vi "Best fit circle.vi"(0 "x array":dbl[](array[numeric]), 1 "y array":dbl[](array[numeric])) -> (2 "x centre":dbl, 3 "y centre":dbl, 4 "radius":dbl)   [LabVIEW 2014]
doc: "Finds the best fit circle using a least squares method. Input arrays (corresponding values of x and y) must have a minimum of 3 values each"
uses:
  <vilib>/Analysis/baseanly.llb/Real A x B.vi
  <vilib>/Analysis/baseanly.llb/A x Vector.vi
  <vilib>/Analysis/baseanly.llb/Real Inverse Matrix.vi
  <vilib>/Analysis/Matrix/Numeric/Conversions/Array To Matrix - RA2.vi
  <vilib>/Analysis/Matrix/NI_Matrix.lvlib
  <vilib>/Analysis/NI_AALBase.lvlib
panel:
  # "Paul Nathan 23/06/2015"
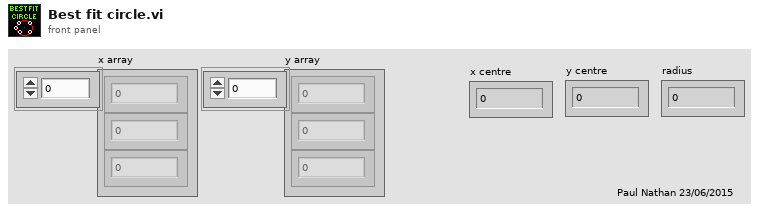
[diagram p1: front panel]
types:
  T1 = typedef "NI_Matrix.lvlib/RealMatrix.ctl" = dbl[][]
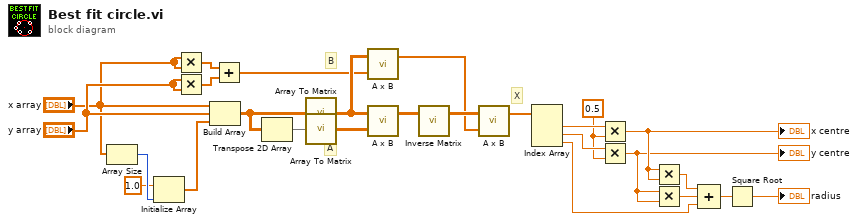
[diagram p0: block diagram]
diagram:
  w8 = 0.5 ("y")
  # "X"
  # "A"
  # "B"
  n1 = Array Size(array="x array") -> (size(s)=w26:i32)
  n2 = Initialize Array(1.0 ("element"), w26) -> (w24:dbl[])
  n3 = Multiply(x="x array", y="x array") -> (x*y=w22:dbl[])
  n4 = Multiply(x="y array", y="y array") -> (x*y=w23:dbl[])
  n5 = Build Array("x array", "y array", w24) -> (w18:dbl[][])
  n6 = Add(x=w22, y=w23) -> (x+y=w12:dbl[])
  n7 = Transpose 2D Array(2D array=w18) -> (transposed array=w19:dbl[][])
  n8 = call-poly <vilib>:"Array To Matrix.vi"("Real 2D Array"=w18) -> ("Real Matrix"=w16:T1)
  n9 = call-poly <vilib>:"Array To Matrix.vi"("Real 2D Array"=w19) -> ("Real Matrix"=w17:T1)
  n10 = call-poly <vilib>:"A x B.vi"("Vector"=w12, "A"=w16) -> ("A x Vector"=w13:dbl[])  [unwired: 1 out]
  n11 = call-poly <vilib>:"A x B.vi"("B"=w17, "A"=w16) -> ("A x B"=w15:T1)  [unwired: 1 out]
  n12 = call-poly <vilib>:"Inverse Matrix.vi"("Input Matrix"=w15) -> ("Inverse Matrix"=w14:T1)  [unwired: 1 in, 1 out]
  n13 = call-poly <vilib>:"A x B.vi"("Vector"=w13, "A"=w14) -> ("A x Vector"=w11:dbl[])  [unwired: 1 out]
  n14 = Index Array(array=w11) -> (element #1=w10:dbl, element #2=w9:dbl, element #3=w3:dbl)  [unwired: 3 in]
  n15 = Multiply(x=w10, y=w8) -> (x*y=w7:dbl)
  "x centre" <- w7
  n16 = Multiply(x=w9, y=w8) -> (x*y=w6:dbl)
  "y centre" <- w6
  n17 = Multiply(x=w7, y=w7) -> (x*y=w5:dbl)
  n18 = Multiply(x=w6, y=w6) -> (x*y=w4:dbl)
  n19 = Compound Arithmetic op=ADD(w5, w4, w3) -> (w2:dbl)
  n20 = Square Root(x=w2) -> (sqrt(x)=→"radius":dbl)
